vi "Excercise2.vi"() -> ()   [LabVIEW 2012]
panel:
  in  "Traditional DAQ Channel":tag
  in  "Deg C":bool
  in  "Temperature":dbl(slide) scale=0.0..10.0
  out "?":dbl
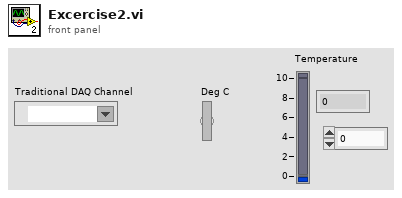
[diagram p1: front panel]
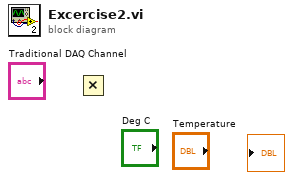
[diagram p0: block diagram]
diagram:
  n1 = Multiply() -> ()  [unwired: 2 in, 1 out]
